vi "Synapse CCD.vi"(8 "error in (no error)":errorcluster) -> (0 "error out":errorcluster, 3 "Synapse CCD.lvclass":refnum<class "Synapse CCD.lvclass">)   [LabVIEW 2009, in "Synapse CCD.lvclass"]
uses:
  Synapse CCD.lvclass
  Global/GPIB Numbers.vi
  Synapse CCD.lvclass/Synapse CCD.ctl
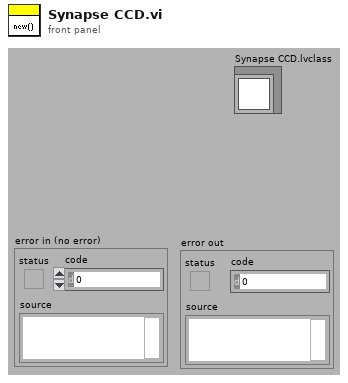
[diagram p1: front panel]
types:
  T1 = typedef "USBCCD Type Def.ctl" = cluster{"Name":string, "Unique ID":string, "Mono Unique ID":string}
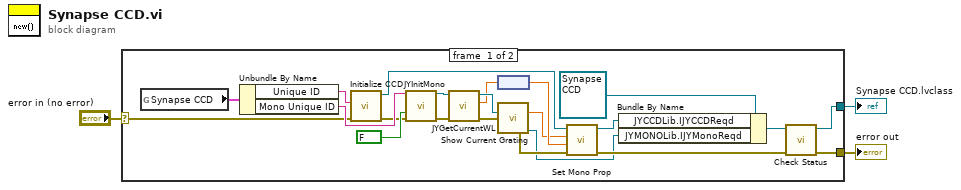
[diagram p0: block diagram]
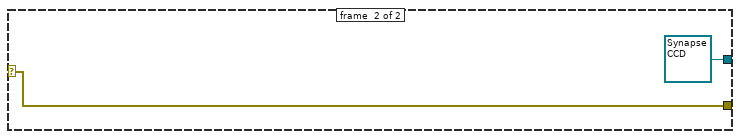
[diagram p2: hidden frame]
diagram:
  n1 = case shown="No Error" "error in (no error)" {
    selector: "error in (no error)" -> [w20 w27]
    tunnel: [w19 refnum<class "Synapse CCD.lvclass"> refnum ("Synapse CCD.lvclass")] -> w3
    tunnel: [w18 w27] -> w2
    frame #0 {
      n2 = global read "GPIB Numbers.vi" "Synapse CCD"() -> (w25:T1)
      n3 = Unbundle By Name(w25) -> ("Unique ID"=w24:string, "Mono Unique ID"=w22:string)
      n4 = call "Initialize CCD.vi"("error in (no error)"=w20, "Unique id:"=w24) -> ("Error out"=w5:errorcluster, "JYCCDLib.IJYCCDReqd Out"=w4:refnum<k7>)  [unwired: 4 in, 4 out]
      n5 = call "JYInitMono.vi"("Unique ID"=w22, "Force Init"=FALSE, "error in (no error)"=w5) -> ("Mono RefNum out"=w13:refnum<k7>, "error out"=w16:errorcluster)  [unwired: 8 in, 3 out]
      n6 = call "JYGetCurrentWL.vi"("error in (no error)"=w16, "JYMONOLib.IJYMonoReqd In"=w13) -> ("error out"=w12:errorcluster, "Current WL"=w10:dbl, "JYMONOLib.IJYMonoReqd Out"=w11:refnum<k7>)  [unwired: 6 in, 1 out]
      n7 = node(w10) -> (w9:dbl[unit])
      n8 = call "Show Current Grating.vi"("JYMONOLib.IJYMonoReqd  in"=w11, "error in (no error)"=w12) -> ("Current Grating"=w8:dbl, "error out"=w7:errorcluster, "JYMONOLib.IJYMonoReqd Out"=w6:refnum<k7>)  [unwired: 5 in, 6 out]
      n9 = call "Set Mono Prop.vi"("error in (no error)"=w7, "Current Wavelength"=w9, "Current Grating"=w8, "IJYCCDReqd In"=w4) -> ("error out"=w15:errorcluster, "IJYCCDReqd out"=w14:refnum<k7>)  [unwired: 6 in]
      n10 = Bundle By Name(cluster=refnum<class "Synapse CCD.lvclass"> refnum ("Synapse CCD.lvclass"), "JYCCDLib.IJYCCDReqd"=w14, "JYMONOLib.IJYMonoReqd"=w6) -> (w21:refnum<class "Synapse CCD.lvclass">)
      n11 = call-dynamic "Check Status.vi"("error in (no error)"=w15, "Synapse CCD in"=w21) -> ("error out"=w18:errorcluster, "Synapse CCD out"=w19:refnum<class "Synapse CCD.lvclass">)  [unwired: 6 in, 2 out]
    }
    frame #1 {
    }
  }
  "Synapse CCD.lvclass" <- w3
  "error out" <- w2
